vi "meas_start_stop.vi"(8 "error in (no error)":errorcluster, 10 "ON/OFF":bool, 11 "Control-Client in":refnum<class "Control-Client.lvclass">) -> (0 "error out":errorcluster, 3 "Control-Client out":refnum<class "Control-Client.lvclass">)   [LabVIEW 2015, in "Control-Client.lvclass"]
uses:
  Control-Client.lvclass
  Control-Client.lvclass/Control-Client.ctl
  GeneralFunctionality/GeneralFunctionality.lvclass/GeneralFunctionality.ctl
  dependecies/XControls/CellsDL/ControlDL.xctl
  controls/Gauge_pump/Gauge_pump.xctl
  Config/Config.lvclass
  GeneralFunctionality/GeneralFunctionality.lvclass
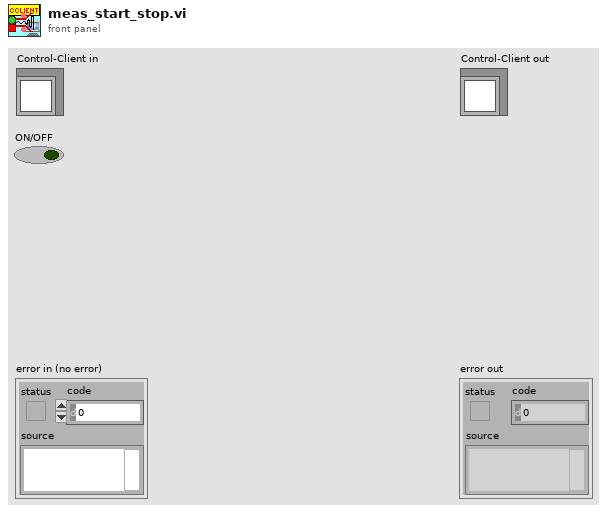
[diagram p1: front panel]
types:
  T1 = typedef "Control-Client.lvclass/Controls-with-permissions_CLIENT.ctl" = cluster{"Server ON/OFF":refnum<vi>, "Detector connect":refnum<vi>, "DL connect":refnum<vi>, "DAQmx connect":refnum<vi>, "All connect":refnum<vi>, "Start measurement":refnum<vi>, "Move Crystal":refnum<vi>, "Relay key heater":refnum<vi>, "Laser Shutter":refnum<vi>, "Accelerator Shutter":refnum<vi>, "Power":refnum<vi>, "Unlock":refnum<vi>, "RT":refnum<vi>, "Faraday Cup":refnum<vi>, "Osc connect":refnum<vi>, "ELYSE pulses":refnum<vi>, "Cells":refnum<vi>, "ControlDL":refnum<vi>, "Pump":refnum<vi>, "# par point":refnum<vi>, "Alarm":refnum<vi>, "oscilloscopeRead":refnum<vi>, "WCM_state":refnum<vi>}
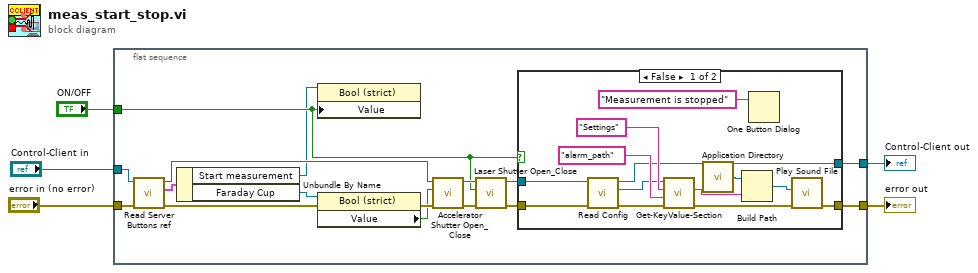
[diagram p0: block diagram]
diagram:
  n1 = flat-sequence {
    tunnel: [w7] -> w5
    tunnel: "Control-Client in" -> [w21]
    tunnel: "error in (no error)" -> [w11]
    tunnel: "ON/OFF" -> [w14]
    tunnel: [w9] -> w1
    frame #0 {
      n2 = call "Read Server Buttons ref.vi"("error in (no error)"=w11, "Control-Client in"=w21) -> ("error out"=w15:errorcluster, "Server Buttons ref"=w20:T1, "Control-Client out"=w12:refnum<class "Control-Client.lvclass">)  [unwired: 7 in]
      n3 = Unbundle By Name(w20) -> ("Start measurement"=w6:refnum<vi>, "Faraday Cup"=w19:refnum<vi>)
      n4 = property class="Bool (strict)"(reference=w6, "Value"=w14) -> ()  [unwired: 1 in, 2 out]
      n5 = property class="Bool (strict)"(reference=w19, error in=w15) -> (error out=w16:errorcluster, "Value"=w13:bool)  [unwired: 1 out]
      n6 = call "Accelerator Shutter Open_Close.vi"("error in (no error)"=w16, "ON/OFF"=w13, "Control-Client in"=w12) -> ("error out"=w17:errorcluster, "Control-Client out"=w18:refnum<class "Control-Client.lvclass">)  [unwired: 7 in]
      n7 = call "Laser Shutter Open_Close.vi"("error in (no error)"=w17, "ON/OFF"=w14, "Control-Client in"=w18) -> ("error out"=w8:errorcluster, "Control-Client out"=w10:refnum<class "Control-Client.lvclass">)  [unwired: 7 in]
      n8 = case shown="False" w14 {
        tunnel: w10 -> [w25 w35]
        tunnel: w8 -> [w24 w36]
        tunnel: [w23 w36] -> w7
        tunnel: [w22 w35] -> w9
        frame False {
          n9 = call "Read Config.vi"("error in (no error)"=w24, "GeneralFunctionality en entrée"=w25) -> ("error out"=w31:errorcluster, "Config.lvclass"=w28:refnum<class "Config.lvclass">, "GeneralFunctionality en sortie"=w22:refnum<class "Control-Client.lvclass">)  [unwired: 7 in]
          n10 = call-dynamic "Get-KeyValue-Section.vi"("error in (no error)"=w31, "Key"="alarm_path", "Section"="Settings", "Config in"=w28) -> ("error out"=w26:errorcluster, "Value"=w27:string)  [unwired: 5 in, 1 out]
          n11 = call <vilib>:"Application Directory.vi"() -> ("Application Directory"=w33:path)
          n12 = Build Path(base path=w33, name or relative path=w27) -> (appended path=w32:path)
          n13 = One Button Dialog(message="Measurement is stopped") -> ()  [unwired: 1 in, 1 out]
          n14 = call <vilib>:"Play Sound File.vi"("error in (no error)"=w26, "path"=w32) -> ("error out"=w23:errorcluster)  [unwired: 8 in, 1 out]
        }
        frame True {
        }
      }
    }
  }
  "error out" <- w5
  "Control-Client out" <- w1
